vi "goToPoint.vi"() -> (0 "y result":dbl, 3 "x result":dbl)   [LabVIEW 2020]
uses:
  <vilib>/Rock Robotics/WPI/ThirdParty/Sensors/navX/_TypeDefs/FRIC_navX_DeviceNumbersTypeDef.ctl
  Robot Global Data.vi
  <vilib>/addons/control/pid/pid.llb/PID (DBL).vi
  <vilib>/addons/control/pid/NI_PID_pid.lvlib
panel:
  in  "y gains":T1={"proportional gain (Kc)"=1.0, "integral time (Ti, min)"=0.01, "derivative time (Td, min)"=0.0} {"derivative time (Td, min)" format="%.25f"; "integral time (Ti, min)" format="%.25f"; "proportional gain (Kc)" format="%.25f"}
  in  "x gains":T1={"proportional gain (Kc)"=1.0, "integral time (Ti, min)"=0.01, "derivative time (Td, min)"=0.0} {"derivative time (Td, min)" format="%.25f"; "integral time (Ti, min)" format="%.25f"; "proportional gain (Kc)" format="%.25f"}
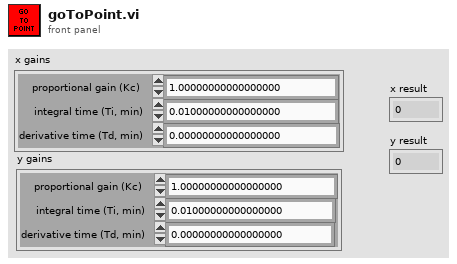
[diagram p1: front panel]
types:
  T1 = cluster{"proportional gain (Kc)":dbl, "integral time (Ti, min)":dbl, "derivative time (Td, min)":dbl}
  T2 = typedef "FRIC_navX_DeviceNumbersTypeDef.ctl" = enum16{"Dev0", "Dev1", "Dev2", "Dev3"}
  T3 = cluster{"Velocity X":dbl, "Velocity Y":dbl, "Velocity Z":dbl, "Displacement X":dbl, "Displacement Y":dbl, "Displacement Z":dbl}
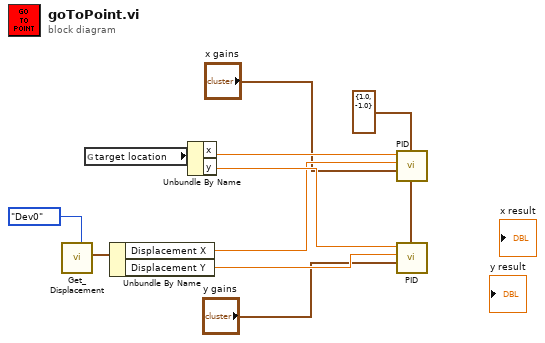
[diagram p0: block diagram]
diagram:
  w8 = cluster{"output high":dbl, "output low":dbl} {"output high"=1.0, "output low"=-1.0} ("output range")
  n1 = call <vilib>:"Get_Displacement.vi"("Device Number"=FRIC_navX_DeviceNumbersTypeDef."Dev0") -> ("Displacement"=w9:T3)  [unwired: 10 in]
  n2 = global read "Robot Global Data.vi" "target location"() -> (w10:cluster{"x":dbl, "y":dbl})
  n3 = Unbundle By Name(w9) -> ("Displacement X"=w5:dbl, "Displacement Y"=w4:dbl)
  n4 = Unbundle By Name(w10) -> ("x"=w7:dbl, "y"=w6:dbl)
  n5 = call-poly <vilib>:"PID.vi"("output range"=w8, "PID gains"="x gains", "process variable"=w5, "setpoint"=w7) -> ()  [unwired: 6 in, 2 out]
  n6 = call-poly <vilib>:"PID.vi"("output range"=w8, "PID gains"="y gains", "process variable"=w4, "setpoint"=w6) -> ()  [unwired: 6 in, 2 out]
